vi "Hormiga_digitalRead.vi"(8 "error in (no error)":errorcluster, 10 "Terminal":u8=13, 11 "VISA Refnum in":refnum<visa-resource-name>) -> (0 "error out":errorcluster, 2 "Returned Value":u8, 3 "VISA Refnum out":refnum<visa-resource-name>)   [LabVIEW 2016]
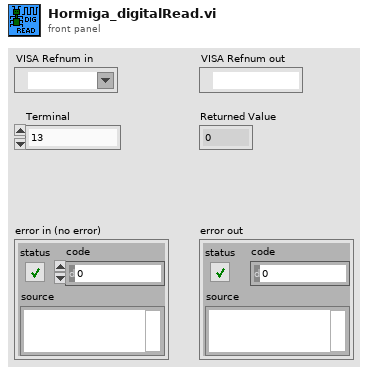
[diagram p1: front panel]
types:
  T1 = enum16{"pinMode", "digitalWrite", "digitalRead", "analogRead", "analogWrite"}
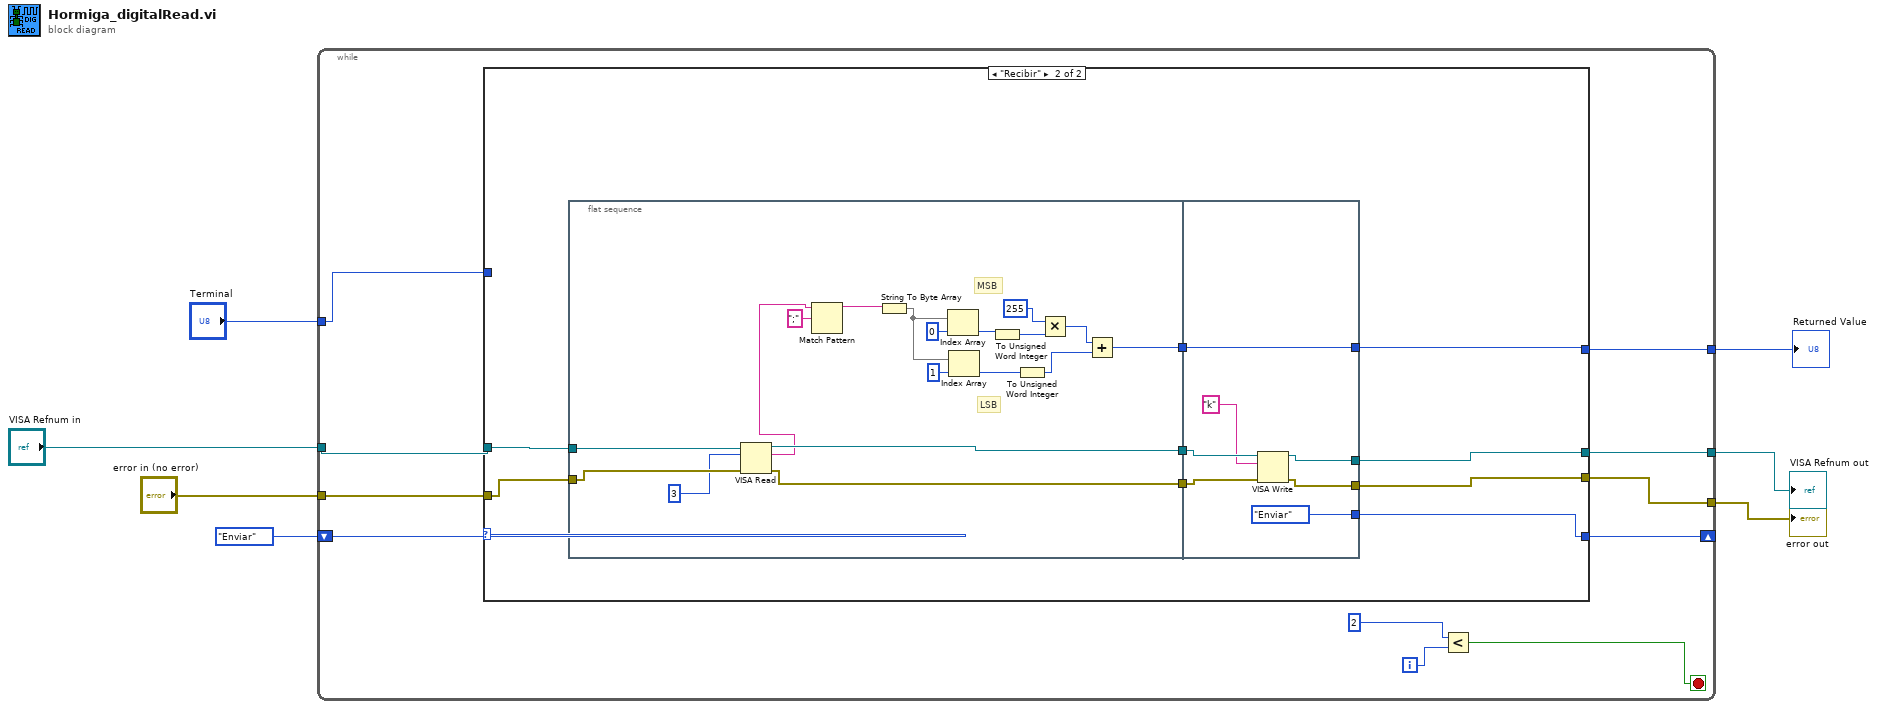
[diagram p0: block diagram]
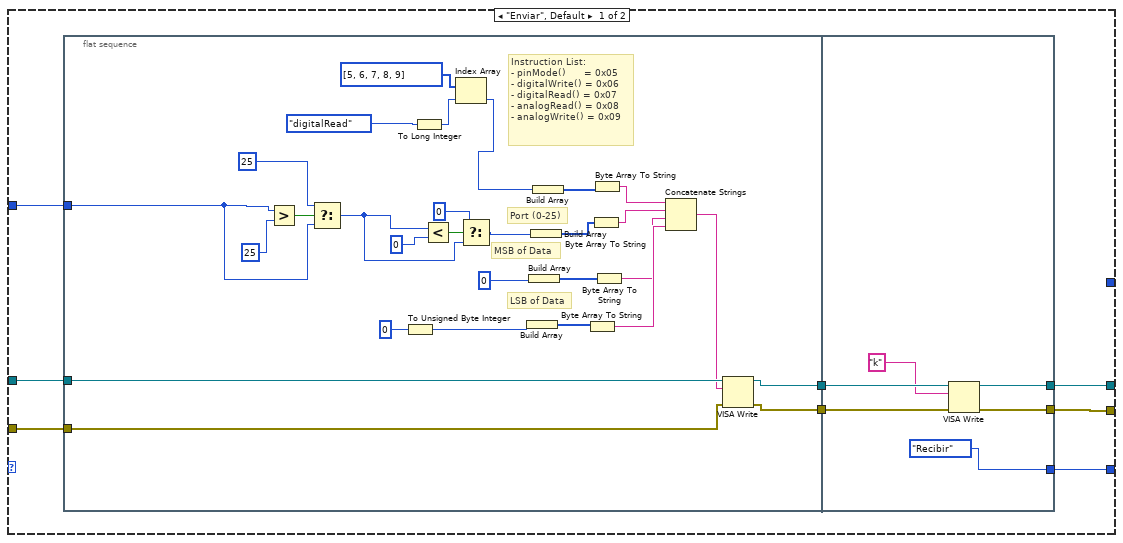
[diagram p2: hidden frame]
diagram:
  n1 = while {
    shift-right: [w13] -> _
    shift-left: enum16{"Enviar", "Recibir"}."Enviar" -> [w18]
    tunnel: "error in (no error)" -> [w17]
    tunnel: "VISA Refnum in" -> [w16]
    tunnel: [w15] -> w3
    tunnel: [w14] -> w4
    tunnel: "Terminal" -> [w9]
    tunnel: [w8] -> w7
    i -> [w11]
    stop <- w12 stop-if-true
    n2 = case shown="\"Recibir\"" w18 {
      tunnel: w17 -> [w26 w70]
      tunnel: w16 -> [w25 w69]
      tunnel: [w22 w66] -> w15
      tunnel: [w21 w65] -> w14
      tunnel: [w20 w64] -> w13
      tunnel: w9 -> [w19 _]
      tunnel: [_ w62] -> w8
      frame "Enviar", Default {
        n3 = flat-sequence {
          tunnel: w26 -> [w55]
          tunnel: w25 -> [w54]
          tunnel: [w53] -> w24
          tunnel: [w52] -> w23
          tunnel: w19 -> [w30]
          tunnel: w24 -> [w61]
          tunnel: w23 -> [w60]
          tunnel: [w58] -> w22
          tunnel: [w57] -> w21
          tunnel: [enum16{"Enviar", "Recibir"}."Recibir"] -> w20
          frame #0 {
            # "Instruction List:\n- pinMode()      = 0x05\n- digitalWrite() = 0x06\n- digitalRead() = 0x07\n- analogRead() = 0x08\n- analogWrite() = 0x09"
            # "LSB of Data"
            # "MSB of Data"
            # "Port (0-25)"
            n4 = Greater?(x=w30, y=u8 25) -> (0:w37:bool)
            n5 = Select(t=u8 25, s=w37, f=w30) -> (s? t:f=w32:u8)
            n6 = To Unsigned Byte Integer(number=u8 0) -> (unsigned 8bit integer=w28:u8)
            n7 = To Long Integer(number=T1."digitalRead") -> (32bit integer=w40:i32)
            n8 = Less?(x=w32, y=u8 0) -> (x < y?=w34:bool)
            n9 = Index Array(array=u8[] [5, 6, 7, 8, 9], index=w40) -> (element=w39:u8)
            n10 = Select(t=u8 0, s=w34, f=w32) -> (s? t:f=w31:u8)
            n11 = Build Array(w28) -> (w47:u8[])
            n12 = Build Array(u8 0) -> (w48:u8[])
            n13 = Build Array(w31) -> (w49:u8[])
            n14 = Build Array(w39) -> (w50:u8[])
            n15 = Byte Array To String(unsigned byte array=w47) -> (string=w46:string)
            n16 = Byte Array To String(unsigned byte array=w49) -> (string=w44:string)
            n17 = Byte Array To String(unsigned byte array=w50) -> (string=w43:string)
            n18 = Byte Array To String(unsigned byte array=w48) -> (string=w45:string)
            n19 = Concatenate Strings(w43, w44, w45, w46) -> (w29:string)
            n20 = VISA Write(VISA resource name=w54, write buffer=w29, error in (no error)=w55) -> (VISA resource name out=w52:refnum<visa-resource-name>, error out=w53:errorcluster)  [unwired: 1 out]
          }
          frame #1 {
            n21 = VISA Write(VISA resource name=w60, write buffer="k", error in (no error)=w61) -> (VISA resource name out=w57:refnum<visa-resource-name>, error out=w58:errorcluster)  [unwired: 1 out]
          }
        }
      }
      frame "Recibir" {
        n22 = flat-sequence {
          tunnel: w70 -> [w80]
          tunnel: w69 -> [w79]
          tunnel: [w88] -> w68
          tunnel: [w87] -> w67
          tunnel: [w81] -> w63
          tunnel: w68 -> [w95]
          tunnel: w67 -> [w94]
          tunnel: [w92] -> w66
          tunnel: [w91] -> w65
          tunnel: [enum16{"Enviar", "Recibir"}."Enviar"] -> w64
          tunnel: w63 -> [w89]
          tunnel: [w89] -> w62
          frame #0 {
            # "MSB"
            # "LSB"
            n23 = VISA Read(VISA resource name=w79, byte count=u32 3, error in (no error)=w80) -> (VISA resource name out=w87:refnum<visa-resource-name>, read buffer=w71:string, error out=w88:errorcluster)  [unwired: 1 out]
            n24 = Match Pattern(string=w71, regular expression=";") -> (before substring=w73:string)  [unwired: 1 in, 3 out]
            n25 = String To Byte Array(string=w73) -> (unsigned byte array=w86:u8[])
            n26 = Index Array(array=w86, index=0) -> (element=w75:u8)
            n27 = Index Array(array=w86, index=1) -> (element=w77:u8)
            n28 = To Unsigned Word Integer(number=w75) -> (unsigned 16bit integer=w74:u16)
            n29 = To Unsigned Word Integer(number=w77) -> (unsigned 16bit integer=w76:u16)
            n30 = Multiply(x=u16 255, y=w74) -> (x*y=w83:u16)
            n31 = Add(x=w83, y=w76) -> (x+y=w81:u16)
          }
          frame #1 {
            n32 = VISA Write(VISA resource name=w94, write buffer="k", error in (no error)=w95) -> (VISA resource name out=w91:refnum<visa-resource-name>, error out=w92:errorcluster)  [unwired: 1 out]
          }
        }
      }
    }
    n33 = Less?(x=2, y=w11) -> (x < y?=w12:bool)
  }
  "Returned Value" <- w7
  "VISA Refnum out" <- w4
  "error out" <- w3
